vi "Actividad_03.vi"() -> ()   [LabVIEW 2025]
panel:
  in  "stop":bool
  in  "Reinicio":bool
  out "Pulsos":dbl
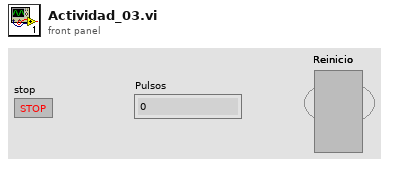
[diagram p1: front panel]
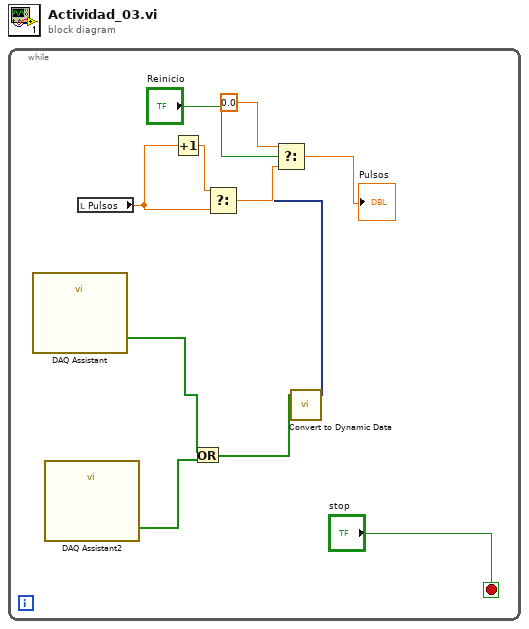
[diagram p0: block diagram]
diagram:
  n1 = while {
    stop <- "stop" stop-if-true
    n2 = call "DAQ Assistant"() -> ("data"=w3:bool[])  [unwired: 17 in, 2 out]
    n3 = call "DAQ Assistant2"() -> ("data"=w2:bool[])  [unwired: 17 in, 2 out]
    n4 = local read "Pulsos"() -> (w11:dbl)
    n5 = Increment(x=w11) -> (x+1=w10:dbl)
    n6 = Or(x=w3, y=w2) -> (x .or. y?=w1:bool[])
    n7 = call "Convert to Dynamic Data"("Array"=w1) -> ("Dynamic Data Type"=w4:dynamicdata)  [unwired: 3 in]
    n8 = Select(t=w10, s=w4, f=w11) -> (s? t:f=w9:dbl)
    n9 = Select(t=0.0, s="Reinicio", f=w9) -> (s? t:f=→"Pulsos":dbl)
  }
